vi "Kalman.vi"(0 "y1":dbl, 5 "y2":dbl, 7 "M":dbl=10.0, 11 "error in (no error)":errorcluster) -> (2 "var1":dbl, 3 "var2":dbl, 4 "y_fused":dbl, 6 "y1":dbl, 8 "y2":dbl, 15 "error out":errorcluster)   [LabVIEW 2017]
panel:
  in  "Tab Control":enum32{"Page 1", "Page 2"}(tab)
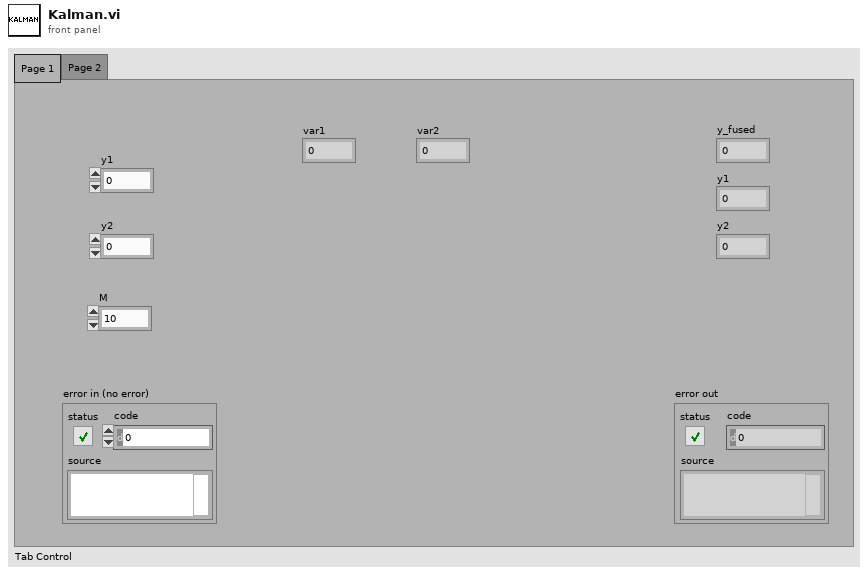
[diagram p1: front panel]
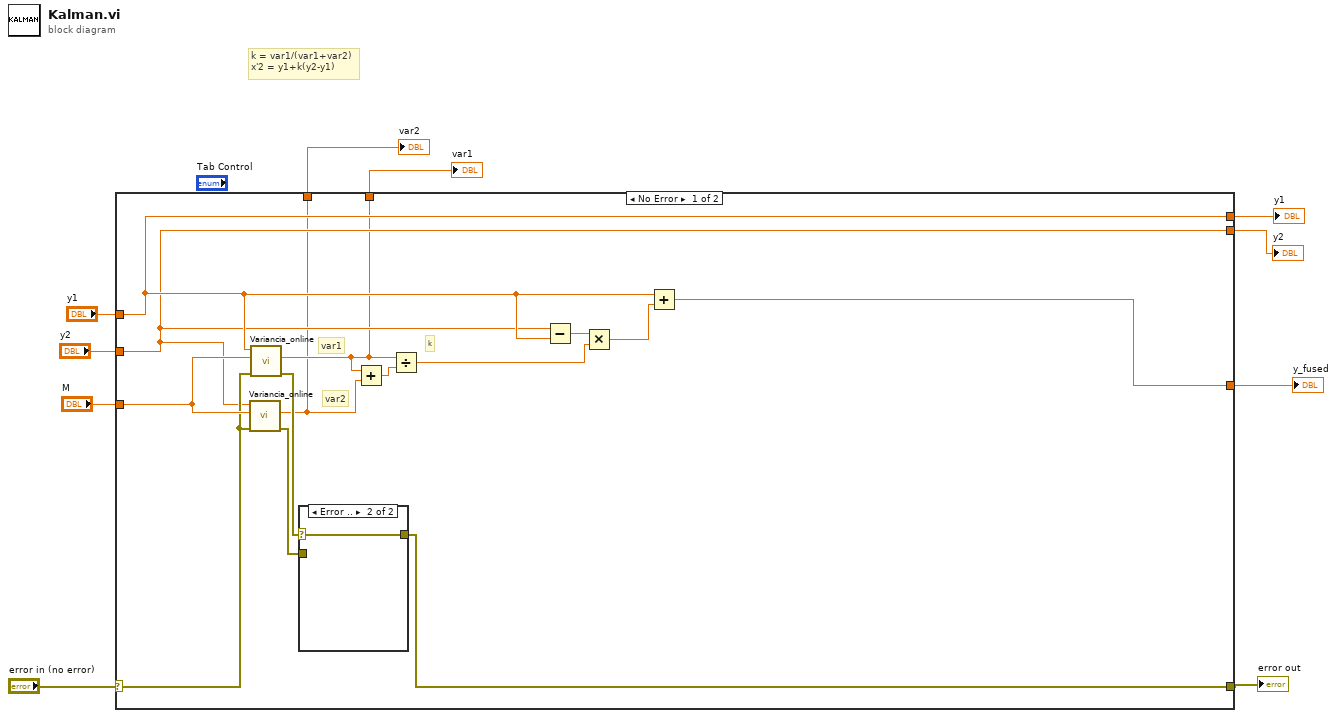
[diagram p0: block diagram]
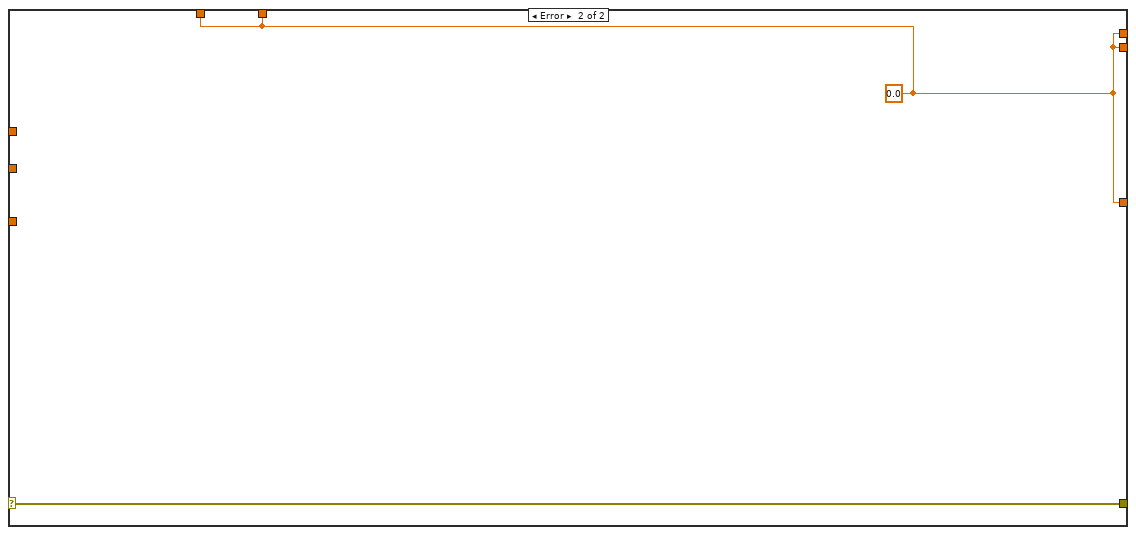
[diagram p4: hidden frame]
diagram:
  # "k = var1/(var1+var2)\nx'2 = y1+k(y2-y1)"
  n1 = case shown="No Error" "error in (no error)" {
    selector: "error in (no error)" -> [w21 w31]
    tunnel: "y2" -> [w17 _]
    tunnel: "y1" -> [w18 _]
    tunnel: [w20 w31] -> w7
    tunnel: [w18 w30] -> w6
    tunnel: [w17 w30] -> w5
    tunnel: "M" -> [w24 _]
    tunnel: [w13 w30] -> w3
    tunnel: [w12 w30] -> w2
    tunnel: [w11 w30] -> w1
    frame No Error {
      # "k"
      # "var2"
      # "var1"
      n2 = call "Variancia_online.vi"("error in (no error)"=w21, "M"=w24, "u"=w17) -> ("error out"=w22:errorcluster, "var"=w11:dbl)  [unwired: 5 in, 2 out]
      n3 = call "Variancia_online.vi"("error in (no error)"=w21, "M"=w24, "u"=w18) -> ("error out"=w23:errorcluster, "var"=w12:dbl)  [unwired: 5 in, 2 out]
      n4 = case shown="Error .." w23 {
        selector: w23 -> [_ w29]
        tunnel: w22 -> [w26 _]
        tunnel: [w25 w29] -> w20
        frame No Error {
          n5 = case shown="Error .." w26 {
            selector: w26 -> [w27 w28]
            tunnel: [w27 w28] -> w25
            frame No Error {
            }
            frame Error {
            }
          }
        }
        frame Error {
        }
      }
      n6 = Add(x=w12, y=w11) -> (x+y=w19:dbl)
      n7 = Divide(x=w12, y=w19) -> (x/y=w15:dbl)
      n8 = Subtract(x=w17, y=w18) -> (x-y=w16:dbl)
      n9 = Multiply(x=w16, y=w15) -> (x*y=w14:dbl)
      n10 = Add(x=w18, y=w14) -> (x+y=w13:dbl)
    }
    frame Error {
      w30 = 0.0
    }
  }
  "y_fused" <- w3
  "error out" <- w7
  "y1" <- w6
  "y2" <- w5
  "var1" <- w2
  "var2" <- w1
